vi "Create Status Log Header.vi"(8 "entrée d'erreur":errorcluster, 11 "Log File Refnum In":refnum<file>) -> (0 "sortie d'erreur":errorcluster, 3 "Log File Refnum out":refnum<file>)   [LabVIEW 2013, in "Logging.lvlib"]
doc: "Ce VI crée l'entête du fichier d'erreur.\nIl classe en colonne : l'heure et la date correspond à la génération de l'erreur , le code de l'erreur, le descriptif de l'erreur."
uses:
  Logging.lvlib
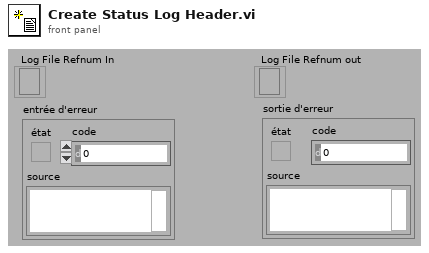
[diagram p1: front panel]
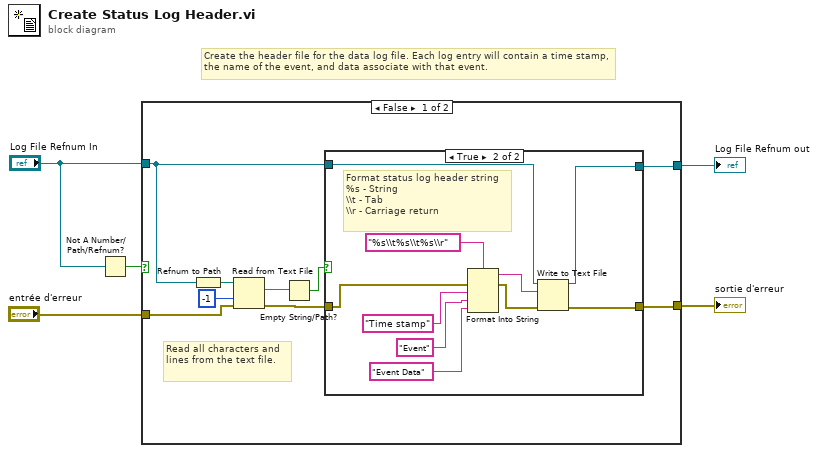
[diagram p0: block diagram]
diagram:
  # "Create the header file for the data log file. Each log entry will contain a time stamp, the name of the event, and data associate with that event."
  n1 = Not A Number/Path/Refnum?(number/path/refnum="Log File Refnum In") -> (NaN/Path/Refnum?=w5:bool)
  n2 = case shown="False" w5 {
    tunnel: "Log File Refnum In" -> [w11 w28]
    tunnel: "entrée d'erreur" -> [w12 w27]
    tunnel: [w10 w28] -> w2
    tunnel: [w8 w27] -> w1
    frame False {
      # "Read all characters and lines from the text file."
      n3 = Refnum to Path(1:w11) -> (0:w14:path)
      n4 = Read from Text File(file (use dialog)=w14, count=-1 ("nombre"), error in=w12) -> (text=w7:string, error out=w9:errorcluster)  [unwired: 1 in, 2 out]
      n5 = Empty String/Path?(string/path=w7) -> (empty?=w6:bool)
      n6 = case shown="True" w6 {
        tunnel: w11 -> [w16 w18]
        tunnel: [w16 w17] -> w10
        tunnel: w9 -> [w15 w23]
        tunnel: [w15 w21] -> w8
        frame False {
        }
        frame True {
          # "Format status log header string\n%s - String\n\\\\t - Tab\n\\\\r - Carriage return"
          n7 = Format Into String(format string="%s\\t%s\\t%s\\r" ("chaîne de format"), error in=w23, "Time stamp", "Event", "Event Data") -> (resulting string=w19:string, error out=w22:errorcluster)  [unwired: 1 in]
          n8 = Write to Text File(file (use dialog)=w18, text=w19, error in=w22) -> (refnum out=w17:refnum<file>, error out=w21:errorcluster)  [unwired: 1 in, 1 out]
        }
      }
    }
    frame True {
    }
  }
  "Log File Refnum out" <- w2
  "sortie d'erreur" <- w1
